vi "getDictDetailsTxt.vi"(8 "error constant":errorcluster, 11 "Dictionary ID Input":string) -> (0 "error IO":errorcluster, 3 "Dictionary":T1)   [LabVIEW 2019]
uses:
  TypeDefs/dictCluster.ctl
  <vilib>/Utility/file.llb/Read Delimited Spreadsheet (string).vi
panel:
  out "all rows":string[][](array[string])
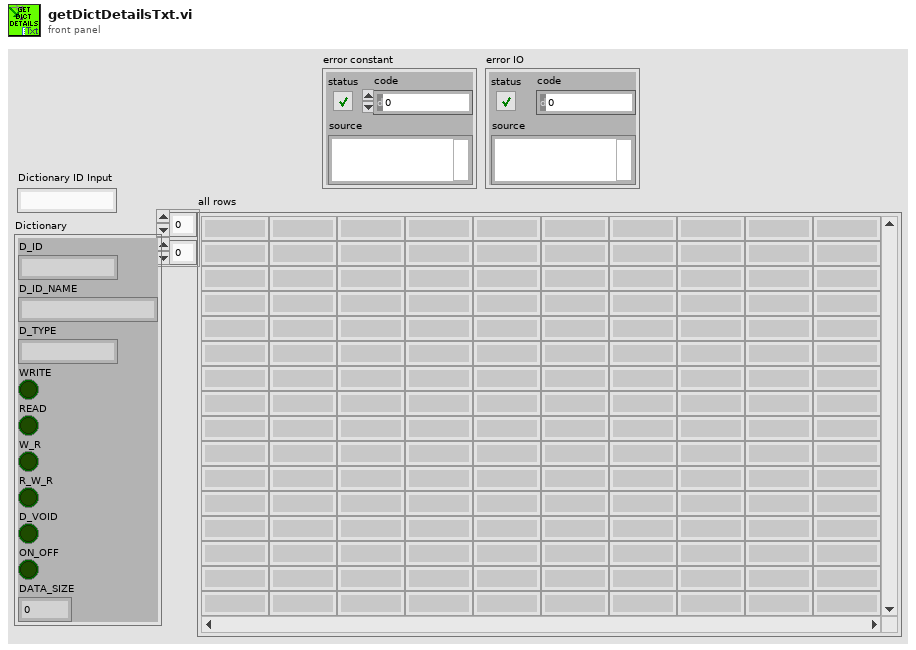
[diagram p1: front panel]
types:
  T1 = cluster{"D_ID":string, "D_ID_NAME":string, "D_TYPE":string, "WRITE":bool, "READ":bool, "W_R":bool, "R_W_R":bool, "D_VOID":bool, "ON_OFF":bool, "DATA_SIZE":u8}
  T2 = typedef "dictCluster.ctl" = cluster{"D_ID":string, "D_ID_NAME":string, "D_TYPE":string, "WRITE":bool, "READ":bool, "W_R":bool, "R_W_R":bool, "D_VOID":bool, "ON_OFF":bool, "DATA_SIZE":u8}
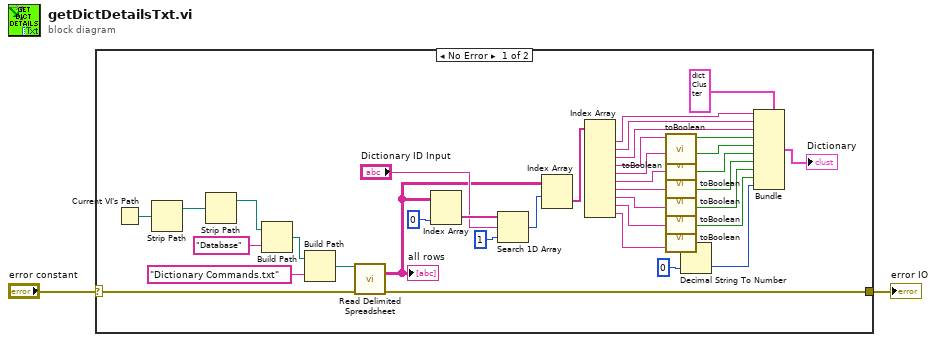
[diagram p0: block diagram]
diagram:
  n1 = case shown="No Error" "error constant" {
    selector: "error constant" -> [w38 w39]
    tunnel: [w30 w39] -> w1
    frame No Error {
      n2 = Current VI's Path() -> (path=w37:path)
      n3 = Strip Path(path=w37) -> (stripped path=w36:path)  [unwired: 1 out]
      n4 = Strip Path(path=w36) -> (stripped path=w35:path)  [unwired: 1 out]
      n5 = Build Path(base path=w35, name or relative path="Database") -> (appended path=w33:path)
      n6 = Build Path(base path=w33, name or relative path="Dictionary Commands.txt") -> (appended path=w31:path)
      n7 = call-poly <vilib>:"Read Delimited Spreadsheet.vi"("file path (dialog if empty)"=w31, "error in (no error)"=w38) -> ("all rows"=w25:string[][], "error out"=w30:errorcluster)  [unwired: 8 in, 4 out]
      "all rows" <- w25
      n8 = Index Array(array=w25, index (col)=0 ("disabled index (col)")) -> (element=w28:string[])  [unwired: 1 in]
      n9 = Search 1D Array(1D array=w28, element="Dictionary ID Input", start index (0)=1) -> (index of element=w24:i32)
      n10 = Index Array(array=w25, index (row)=w24) -> (element=w22:string[])  [unwired: 1 in]
      n11 = Index Array(array=w22) -> (element #1=w21:string, element #2=w20:string, element #3=w19:string, element #4=w18:string, element #5=w16:string, element #6=w15:string, element #7=w14:string, element #8=w13:string, element #9=w12:string, element #10=w11:string)  [unwired: 10 in]
      n12 = call "toBoolean.vi"("String"=w18) -> ("Boolean"=w17:bool)  [unwired: 10 in]
      n13 = call "toBoolean.vi"("String"=w16) -> ("Boolean"=w4:bool)  [unwired: 10 in]
      n14 = call "toBoolean.vi"("String"=w15) -> ("Boolean"=w5:bool)  [unwired: 10 in]
      n15 = call "toBoolean.vi"("String"=w14) -> ("Boolean"=w6:bool)  [unwired: 10 in]
      n16 = call "toBoolean.vi"("String"=w13) -> ("Boolean"=w7:bool)  [unwired: 10 in]
      n17 = call "toBoolean.vi"("String"=w12) -> ("Boolean"=w8:bool)  [unwired: 10 in]
      n18 = Decimal String To Number(string=w11, default (0L)=u8 0 ("default (0 I32)")) -> (number=w9:u8)  [unwired: 1 in, 1 out]
      n19 = Bundle(cluster=T2 {"D_ID"="", "D_ID_NAME"="", "D_TYPE"="", "WRITE"=FALSE, "READ"=FALSE, "W_R"=FALSE, "R_W_R"=FALSE, "D_VOID"=FALSE, "ON_OFF"=FALSE, "DATA_SIZE"=0} ("Dictionary"), "D_ID"=w21, "D_ID_NAME"=w20, "D_TYPE"=w19, "WRITE"=w17, "READ"=w4, "W_R"=w5, "R_W_R"=w6, "D_VOID"=w7, "ON_OFF"=w8, "DATA_SIZE"=w9) -> (→"Dictionary":T2)
    }
    frame Error {
    }
  }
  "error IO" <- w1
